vi "errorcodehandler.vi"(2 "show description (T)":bool=TRUE, 3 "show DLL error code (F)":bool, 4 "show name (F)":bool, 5 "error cluster":errorcluster) -> (0 "code":i32, 1 "description":string)   [LabVIEW 2011]
doc: "Looks up an error description string from an <B>error cluster</B> obtained from an SDK SubVI. The error cluster's <B>code</B> member is also returned (for conveniency)."
uses:
  lib/atmcd32d.llb/Error Code Enum typedef.ctl
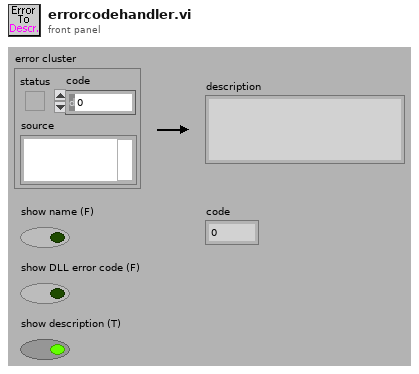
[diagram p1: front panel]
types:
  T1 = typedef "Error Code Enum typedef.ctl" = enum32{"N/A (0)", "DRV_ERROR_CODES", "DRV_SUCCESS", "DRV_VXDNOTINSTALLED", "DRV_ERROR_SCAN", "DRV_ERROR_CHECK_SUM", "DRV_ERROR_FILELOAD", "DRV_UNKNOWN_FUNC", "DRV_ERROR_VXD_INIT", "DRV_ERROR_ADDRESS", "DRV_ERROR_PAGELOCK", "DRV_ERROR_PAGEUNLOCK", "DRV_ERROR_BOARDTEST", "DRV_ERROR_ACK", "DRV_ERROR_UP_FIFO", "DRV_ERROR_PATTERN", "N/A (16)", "DRV_ACQUISITION_ERRORS", "DRV_ACQ_BUFFER", "DRV_ACQ_DOWNFIFO_FULL", "DRV_PROC_UNKONWN_INSTRUCTION", "DRV_ILLEGAL_OP_CODE", "DRV_KINETIC_TIME_NOT_MET", "DRV_ACCUM_TIME_NOT_MET", "DRV_NO_NEW_DATA", "N/A (25)", "DRV_SPOOLERROR", "N/A (27)", "N/A (28)", "N/A (29)", "N/A (30)", "N/A (31)", "N/A (32)", "DRV_TEMPERATURE_CODES", "DRV_TEMPERATURE_OFF", "DRV_TEMPERATURE_NOT_STABILIZED", "DRV_TEMPERATURE_STABILIZED", "DRV_TEMPERATURE_NOT_REACHED", "DRV_TEMPERATURE_OUT_RANGE", "DRV_TEMPERATURE_NOT_SUPPORTED", "DRV_TEMPERATURE_DRIFT", "N/A (41)", "N/A (42)", "N/A (43)", "N/A (44)", "N/A (45)", "N/A (46)", "N/A (47)", "N/A (48)", "DRV_GENERAL_ERRORS", "DRV_INVALID_AUX", "DRV_COF_NOTLOADED", "DRV_FPGAPROG", "DRV_FLEXERROR", "DRV_GPIBERROR", "N/A (55)", "N/A (56)", "N/A (57)", "N/A (58)", "N/A (59)", "N/A (60)", "N/A (61)", "N/A (62)", "N/A (63)", "DRV_DATATYPE", "DRV_DRIVER_ERRORS", "DRV_P1INVALID", "DRV_P2INVALID", "DRV_P3INVALID", "DRV_P4INVALID", "DRV_INIERROR", "DRV_COFERROR", "DRV_ACQUIRING", "DRV_IDLE", "DRV_TEMPCYCLE", "DRV_NOT_INITIALIZED", "DRV_P5INVALID", "DRV_P6INVALID", "DRV_INVALID_MODE", "DRV_INVALID_FILTER", "DRV_I2CERRORS", "DRV_I2CDEVNOTFOUND", "DRV_I2CTIMEOUT", "DRV_P7INVALID", "N/A (84)", "N/A (85)", "N/A (86)", "N/A (87)", "N/A (88)", "N/A (89)", "DRV_IOCERROR", "DRV_VRMVERSIONERROR"}
  T2 = typedef "Function Enum typedef.ctl" = enum8{"N/A (0)", "AbortAcquisition", "CoolerOFF", "CoolerON", "FreeInternalMemory", "GetAcquiredData", "GetAcquiredData16", "GetAcquisitionProgress", "GetAcquisitionTimings", "GetCapabilities", "GetDDGIOCPulses", "GetDDGPulse", "GetDetector", "GetFilterMode", "GetFKExposureTime", "GetFKVShiftSpeedF", "GetHardwareVersion", "GetHeadModel", "GetHSSpeed", "GetNewData", "GetNewData16", "GetNumberADChannels", "GetNumberAmp", "GetNumberFKVShiftSpeeds", "GetNumberHSSpeeds", "GetNumberPreAmpGains", "GetNumberVSSpeeds", "GetPixelSize", "GetPreAmpGain", "GetSoftwareVersion", "GetStatus", "GetTemperature", "GetTemperatureRange", "GetVSSpeed", "GPIBReceive", "GPIBSend", "I2CBurstRead", "I2CBurstWrite", "I2CRead", "I2CReset", "I2CWrite", "InAuxPort", "Initialize", "OutAuxPort", "PrepareAcquisition", "SaveAsBmp", "SaveAsCommentedSif", "SaveAsSif", "SaveAsTiff", "SetAccumulationCycleTime", "SetAcquisitionMode", "SetADChannel", "SetBaselineClamp", "SetCustomTrackHBin", "SetDDGGain", "SetDDGGateStep", "SetDDGInsertionDelay", "SetDDGIntelligate", "SetDDGIOC", "SetDDGIOCFrequency", "SetDDGTimes", "SetDDGTriggerMode", "SetDDGVariableGateStep", "SetDelayGenerator", "SetDriverEvent", "SetEMCCDGain", "SetExposureTime", "SetFanMode", "SetFastExtTrigger", "SetFastKinetics", "SetFastKineticsEx", "SetFilterMode", "SetFKVShiftSpeed", "SetFullImage", "SetFVBHBin", "SetGain", "SetGate", "SetGateMode", "SetHSSpeed", "SetImage", "SetKineticCycleTime", "SetMCPGating", "SetMultiTrack", "SetMultiTrackHBin", "SetNumberAccumulations", "SetNumberKinetics", "SetOutputAmplifier", "SetPhotonCounting", "SetPhotonCountingThreshold", "SetPreAmpGain", "SetRandomTracks", "SetReadMode", "SetShutter", "SetSifComment", "SetSingleTrack", "SetSingleTrackHBin", "SetSpool", "SetTemperature", "SetTriggerMode", "SetVSAmplitude", "SetVSSpeed", "ShutDown", "StartAcquisition"}
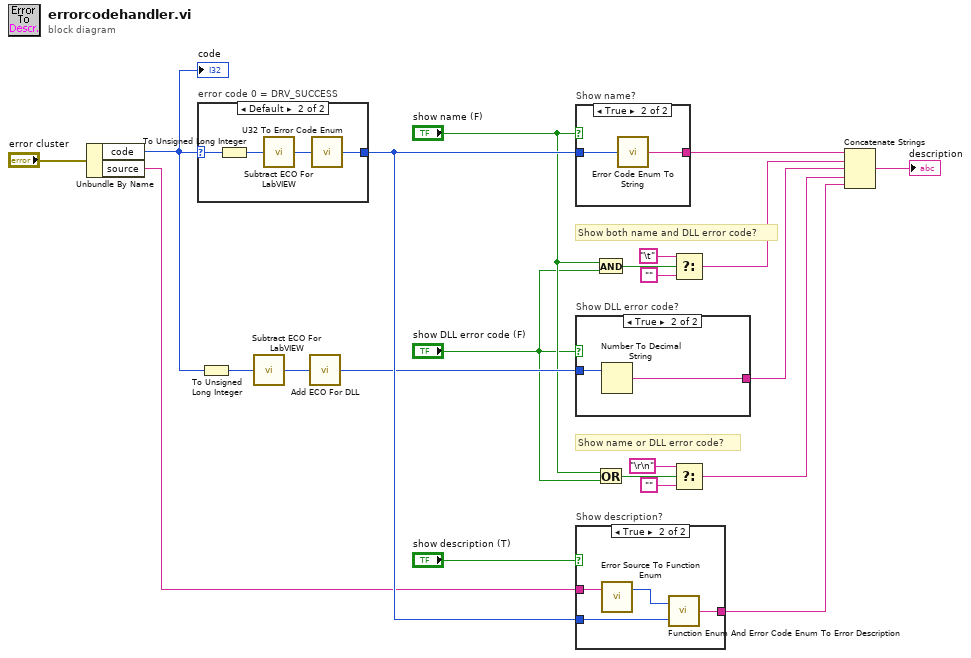
[diagram p0: block diagram]
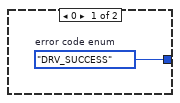
[diagram p5: hidden frame]
diagram:
  # "Show name or DLL error code?"
  # "Show both name and DLL error code?"
  n1 = Unbundle By Name("error cluster") -> ("code"=w9:i32, "source"=w18:string)
  "code" <- w9
  n2 = case "error code 0 = DRV_SUCCESS" shown="Default" w9 {
    selector: w9 -> [_ w24]
    tunnel: [w23 w25] -> w20
    frame 0 {
      w23 = Error_Code_Enum_typedef."DRV_SUCCESS"  # error code enum
    }
    frame Default {
      n3 = To Unsigned Long Integer(number=w24) -> (unsigned 32bit integer=w27:u32)
      n4 = call "Subtract ECO For LabVIEW.vi"("x"=w27) -> ("x - ECO4LabVIEW"=w26:u32)
      n5 = call "U32 To Error Code Enum.vi"("U32"=w26) -> ("error code enum"=w25:T1)
    }
  }
  n6 = To Unsigned Long Integer(number=w9) -> (unsigned 32bit integer=w8:u32)
  n7 = call "Subtract ECO For LabVIEW.vi"("x"=w8) -> ("x - ECO4LabVIEW"=w11:u32)
  n8 = call "Add ECO For DLL.vi"("x"=w11) -> ("x + ECO4DLL"=w10:u32)
  n9 = case "Show name?" shown="True" "show name (F)" {
    tunnel: w20 -> [_ w29]
    tunnel: [_ w28] -> w3
    frame False {
    }
    frame True {
      n10 = call "Error Code Enum To String.vi"("error code enum"=w29) -> ("string"=w28:string)
    }
  }
  n11 = case "Show DLL error code?" shown="True" "show DLL error code (F)" {
    tunnel: w10 -> [_ w31]
    tunnel: [_ w30] -> w17
    frame False {
    }
    frame True {
      n12 = Number To Decimal String(number=w31) -> (decimal integer string=w30:string)  [unwired: 1 in]
    }
  }
  n13 = case "Show description?" shown="True" "show description (T)" {
    tunnel: w20 -> [_ w35]
    tunnel: w18 -> [_ w34]
    tunnel: [_ w32] -> w13
    frame False {
    }
    frame True {
      n14 = call "Error Source To Function Enum.vi"("error source"=w34) -> ("function enum"=w33:T2)  [unwired: 1 in, 1 out]
      n15 = call "Function Enum And Error Code Enum To Error Description.vi"("error code enum"=w35, "function enum"=w33) -> ("error description"=w32:string)
    }
  }
  n16 = And(x="show name (F)", y="show DLL error code (F)") -> (x .and. y?=w6:bool)
  n17 = Or(x="show name (F)", y="show DLL error code (F)") -> (x .or. y?=w16:bool)
  n18 = Select(t="\t", s=w6, f="") -> (s? t:f=w2:string)
  n19 = Select(t="\r\n", s=w16, f="") -> (s? t:f=w12:string)
  n20 = Concatenate Strings(w3, w2, w17, w12, w13) -> (→"description":string)
